vi "array_loops.vi"(10 "values_IN":dbl[](array[numeric])=[1.0, 2.0, 3.0, 4.0, 5.0, 6.0, 7.0, 8.0, 9.0, 10.0] format="%#_6p", 11 "loops":i32=1 min=0) -> (2 "values_OUT":dbl[](array[numeric])=[1.0, 2.0, 3.0, 4.0, 5.0, 6.0, 7.0, 8.0, 9.0, 10.0] format="%#_6p")   [LabVIEW 2017, in "tools.lvlib"]
uses:
  tools.lvlib
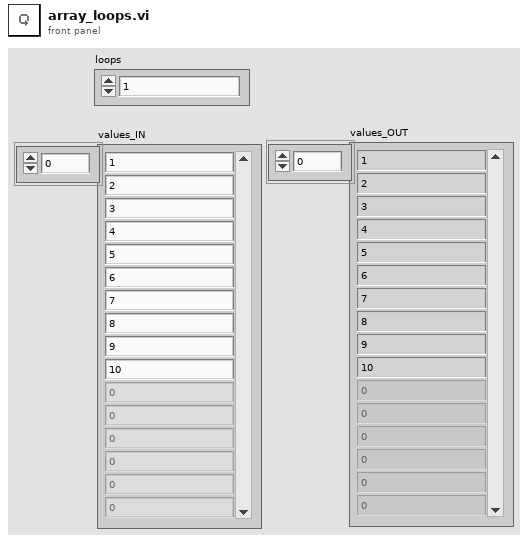
[diagram p1: front panel]
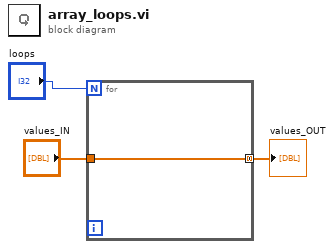
[diagram p0: block diagram]
diagram:
  n1 = for {
    N: "loops" -> [_]
    tunnel: "values_IN" -> [w4]
    tunnel: [w4] -> w2 mode=concatenating
  }
  "values_OUT" <- w2
